vi "ABCD lens.vi"(1 "Focal length":dbl format="%.2f") -> (0 "ABCD":cluster{"A":dbl, "B":dbl, "C":dbl, "D":dbl} {"D" format="%.2f"; "C" format="%.2f"; "B" format="%.2f"; "A" format="%.2f"})   [LabVIEW 2016]
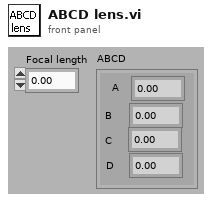
[diagram p1: front panel]
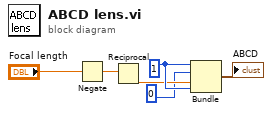
[diagram p0: block diagram]
diagram:
  w5 = 1
  n1 = Negate(x="Focal length") -> (-x=w1:dbl)
  n2 = Reciprocal(x=w1) -> (1/x=w4:dbl)
  n3 = Bundle(w5, "Index (row)"=0, w4, w5) -> (→"ABCD":cluster{i32, "Index (row)":i32, dbl, i32})  [unwired: 1 in]
